vi "split_and_queue_string_at_front.vi"(8 "error in (no error)":errorcluster, 10 "program string":string, 11 "queue in":refnum<queue>) -> (0 "error out":errorcluster, 3 "queue out":refnum<queue>)   [LabVIEW 2015]
panel:
  # "Split & queue string at front"
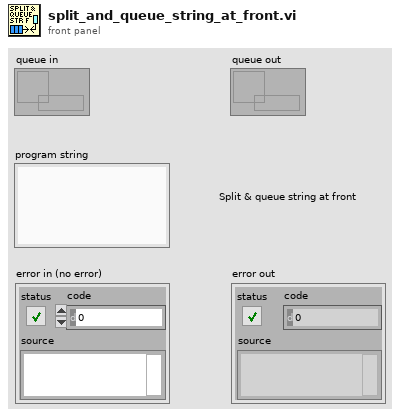
[diagram p1: front panel]
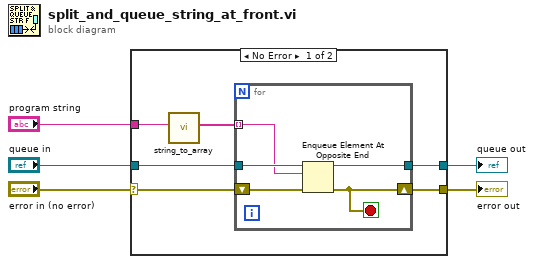
[diagram p0: block diagram]
diagram:
  n1 = case shown="No Error" "error in (no error)" {
    selector: "error in (no error)" -> [w10 w18]
    tunnel: [w9 w18] -> w1
    tunnel: "program string" -> [w11 _]
    tunnel: "queue in" -> [w8 w17]
    tunnel: [w7 w17] -> w2
    frame No Error {
      n2 = call "string_to_array.vi"("program string"=w11) -> ("array"=w6:string[])  [unwired: 10 in]
      n3 = for {
        shift-right: [w12] -> w9
        shift-left: w10 -> [w16]
        tunnel: w8 -> [w15]
        tunnel: [w14] -> w7
        tunnel: w6 -> [w13] mode=indexing
        stop <- w12 stop-if-true
        n4 = Enqueue Element At Opposite End(queue=w15, element=w13, error in (no error)=w16) -> (queue out=w14:refnum<queue>, error out=w12:errorcluster)  [unwired: 1 in, 1 out]
      }
    }
    frame Error {
    }
  }
  "error out" <- w1
  "queue out" <- w2
